vi "checkBeginPreparePassPlay.vi"(8 "error in (no error)":errorcluster, 10 "Game":refnum<class "Game.lvclass">, 11 "PreparePassPlay in":refnum<class "PreparePassPlay.lvclass">) -> (0 "error out":errorcluster, 2 "Boolean":bool, 3 "PreparePassPlay out":refnum<class "PreparePassPlay.lvclass">)   [LabVIEW 2018, in "PreparePassPlay.lvclass"]
uses:
  PreparePassPlay.lvclass
  Game_class/Game.lvclass
  Game_class/Game.lvclass/Game.ctl
  Referee_class/Referee.lvclass/Referee.ctl
  Referee_class/command_interpreted.ctl
  Game_class/Read Referee.vi
  Referee_class/Read command_interpreted.vi
  Referee_class/Referee.lvclass
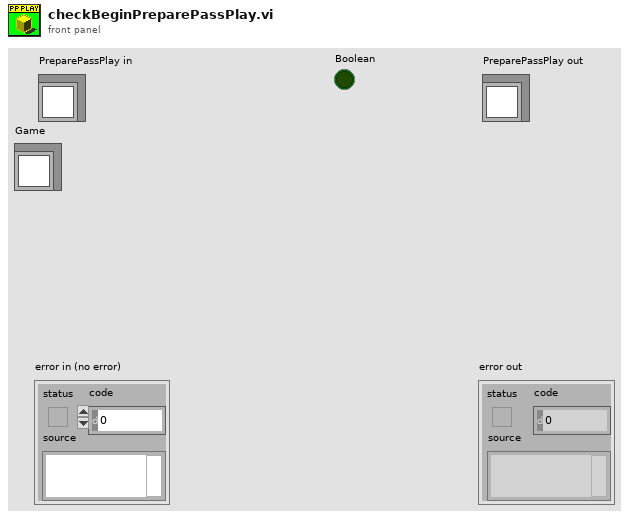
[diagram p1: front panel]
types:
  T1 = typedef "command_interpreted.ctl" = enum16{"Goal Ally", "Goal Enemy", "Ball Placement Enemy", "Ball Placement Ally", "Normal Half Time", "Extra Time  Break", "Extra Half Time", "None", "Post Game", "PKA Normal Start", "Prepare Kickoff Ally", "PKE Normal Start", "Prepare Kickoff Enemy", "Force Start", "Halt", "Timeout", "Prepare Penalty Ally", "Prepare Penalty Enemy", "PPA NormalStart", "PPE Normal Start", "Indirect Free Ally", "Direct Free Enemy", "Direct Free Ally", "Indirect Free Enemy", "Stop"}
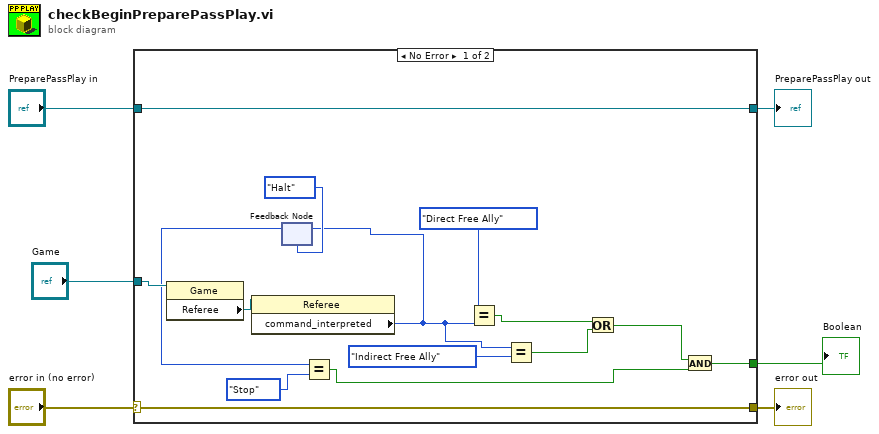
[diagram p0: block diagram]
diagram:
  n1 = case shown="No Error" "error in (no error)" {
    selector: "error in (no error)" -> [w20 w23]
    tunnel: [w20 w23] -> w5
    tunnel: [w21 w22] -> w3
    tunnel: "PreparePassPlay in" -> [w21 w22]
    tunnel: "Game" -> [w19 _]
    tunnel: [w15 _] -> w1
    frame No Error {
      n2 = property class="Game"(reference=w19) -> ("Referee"=w18:refnum<class "Referee.lvclass">)  [unwired: 1 in, 2 out]
      n3 = property class="Referee"(reference=w18) -> ("command_interpreted"=w7:T1)  [unwired: 1 in, 2 out]
      n4 = feedback-in #1(w7) -> ()
      n5 = feedback #1(command_interpreted."Halt" ("command_interpreted")) -> (w17:T1)
      n6 = Equal?(x=w17, y=command_interpreted."Stop" ("command_interpreted")) -> (x = y?=w14:bool)
      n7 = Equal?(x=command_interpreted."Direct Free Ally" ("command_interpreted"), y=w7) -> (x = y?=w11:bool)
      n8 = Equal?(x=w7, y=command_interpreted."Indirect Free Ally" ("command_interpreted")) -> (x = y?=w10:bool)
      n9 = Or(x=w11, y=w10) -> (x .or. y?=w9:bool)
      n10 = And(x=w9, y=w14) -> (x .and. y?=w15:bool)
    }
    frame Error {
    }
  }
  "error out" <- w5
  "PreparePassPlay out" <- w3
  "Boolean" <- w1
